vi "Generate CSM Class mermaid.vi"(8 "error in (no error)":errorcluster, 11 "VI":refnum<vi>) -> (0 "error out":errorcluster, 3 "resulting string":string)   [LabVIEW 2020]
uses:
  <userlib>/_NEVSTOP/Communicable State Machine(CSM)/Communicable State Machine.lvlib
  CSM-Helper/CSM-Helper.lvclass
  CSM-Helper/Properties/Read User-Defined States.vi
  CSM-Helper/API/Create From VI Reference.vi
  CSM-Helper/API/Destroy.vi
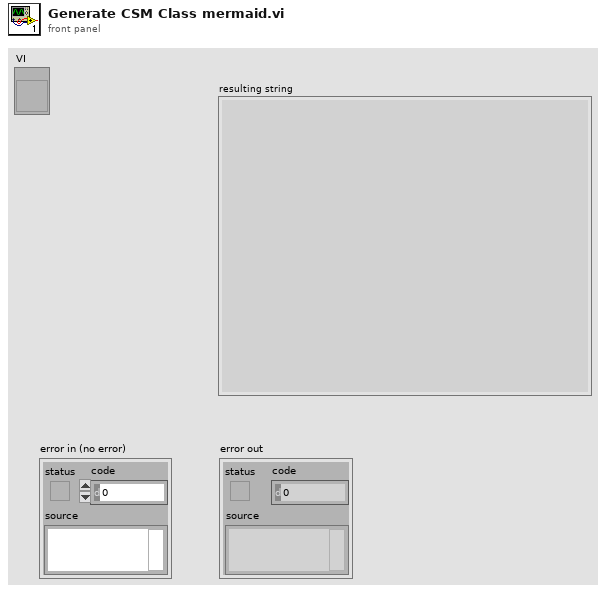
[diagram p1: front panel]
types:
  T1 = typedef "CSM-Helper.lvclass/Def-Argument Info.ctl" = cluster{"Type":string, "Name":string, "Variant":variant}
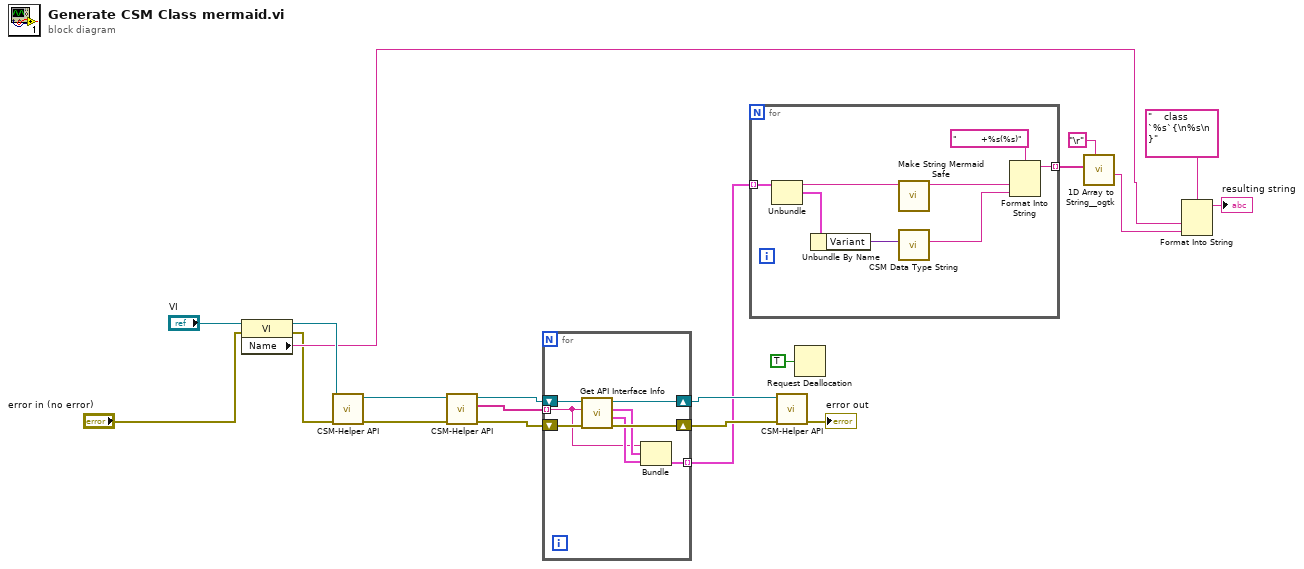
[diagram p0: block diagram]
diagram:
  n1 = property class="VI"(reference="VI", error in="error in (no error)") -> (reference out=w4:refnum<vi>, error out=w1:errorcluster, "Name"=w3:string)
  n2 = call-poly "CSM-Helper API.vi"("error in (no error)"=w1, "VI"=w4) -> ("error out"=w20:errorcluster, "CSM-Helper.lvclass"=w14:refnum<class "CSM-Helper.lvclass">)  [unwired: 8 in]
  n3 = call-poly "CSM-Helper API.vi"("error in (no error)"=w20, "CSM-Helper in"=w14) -> ("error out"=w13:errorcluster, "Array"=w9:string[], "CSM-Helper out"=w12:refnum<class "CSM-Helper.lvclass">)  [unwired: 7 in]
  n4 = for {
    shift-right: [w25] -> w10
    shift-left: w13 -> [w28]
    shift-right: [w26] -> w11
    shift-left: w12 -> [w27]
    tunnel: w9 -> [w21] mode=indexing
    tunnel: [w22] -> w8 mode=indexing
    n5 = call "Get API Interface Info.vi"("error in (no error)"=w28, "CASE"=w21, "CSM-Helper in"=w27) -> ("error out"=w25:errorcluster, "Response"=w24:T1, "Argument"=w23:T1, "CSM-Helper out"=w26:refnum<class "CSM-Helper.lvclass">)  [unwired: 5 in]
    n6 = Bundle(w21, "Argument"=w23, "Response"=w24) -> (w22:cluster{string, "Argument":T1, "Response":T1})  [unwired: 1 in]
  }
  n7 = for {
    tunnel: [w35] -> w19 mode=indexing
    tunnel: w8 -> [w33] mode=indexing
    n8 = Unbundle(w33) -> (w32:string, "Argument"=w31:T1)  [unwired: 1 out]
    n9 = Unbundle By Name(w31) -> ("Variant"=w30:variant)
    n10 = call "Make String Mermaid Safe.vi"("Source CSM"=w32) -> ("result string"=w34:string)  [unwired: 10 in]
    n11 = call <userlib>:"CSM Data Type String.vi"("Data"=w30) -> ("Data Type String"=w29:string)  [unwired: 10 in]
    n12 = Format Into String(format string="        +%s(%s)", w34, w29) -> (resulting string=w35:string)  [unwired: 2 in, 1 out]
  }
  n13 = call-poly "CSM-Helper API.vi"("error in (no error)"=w10, "CSM-Helper in"=w11) -> ("error out"=→"error out":errorcluster)  [unwired: 8 in, 1 out]
  n14 = Request Deallocation(TRUE ("flag")) -> ()
  n15 = call <userlib>:"1D Array to String__ogtk.vi"("delimiter (Tab)"="\r", "Array of Strings"=w19) -> ("delimited string"=w15:string)  [unwired: 9 in]
  n16 = Format Into String(format string="    class `%s`{\n%s\n    }", w3, w15) -> (resulting string=→"resulting string":string)  [unwired: 2 in, 1 out]
